vi "Inner Measure.vi"(8 "error in (no error)":errorcluster, 11 "Measurement3D in":refnum<class "Measurement3D.lvclass">) -> (0 "error out":errorcluster, 1 "Current Value":dbl, 2 "Result":dbl, 3 "Measurement3D out":refnum<class "Measurement3D.lvclass">)   [LabVIEW 2014, in "Measurement3D.lvclass"]
uses:
  Measurement3D.lvclass
  Instrument/Instrument/Instrument.lvclass
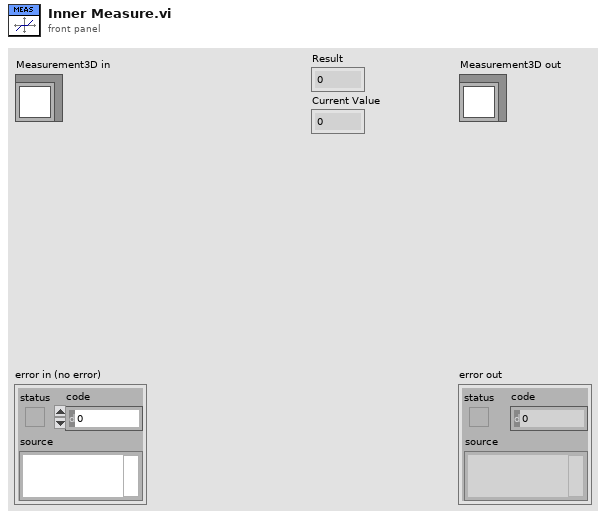
[diagram p1: front panel]
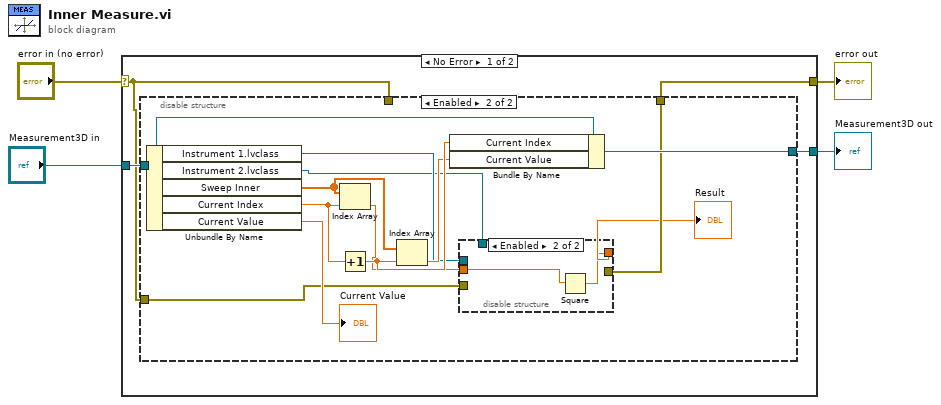
[diagram p0: block diagram]
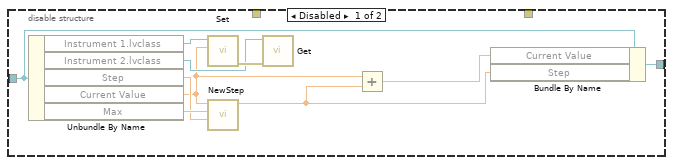
[diagram p2: hidden frame]
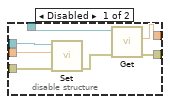
[diagram p3: hidden frame]
diagram:
  n1 = case shown="No Error" "error in (no error)" {
    selector: "error in (no error)" -> [w5 w42]
    tunnel: [w6 w42] -> w3
    tunnel: [w7 w41] -> w1
    tunnel: "Measurement3D in" -> [w8 w41]
    frame No Error {
      n2 = disable-structure shown="Enabled" {
        disable-tunnel: w8 -> [w12 w26]
        disable-tunnel: [w9 w25] -> w7
        disable-tunnel: w5 -> [_ _]
        disable-tunnel: [_ w20] -> w6
        disable-tunnel: w5 -> [_ w24]
        frame Disabled {
          n3 = Unbundle By Name(w12) -> ("Instrument 1.lvclass"=w18:refnum<class "Instrument.lvclass">, "Instrument 2.lvclass"=w14:refnum<class "Instrument.lvclass">, "Step"=w15:dbl, "Current Value"=w13:dbl, "Max"=w16:dbl)
          n4 = call-dynamic "Set.vi"("Numeric"=w13, "Instrument in"=w18) -> ("error out"=w17:errorcluster)  [unwired: 8 in, 1 out]
          n5 = call "NewStep.vi"("Step"=w15, "Max"=w16, "Current Value"=w13) -> ("Step 2"=w10:dbl)  [unwired: 8 in]
          n6 = call-dynamic "Get.vi"("error in (no error)"=w17, "Instrument in"=w14) -> ()  [unwired: 7 in, 3 out]
          n7 = Add(x=w13, y=w10) -> (x+y=w11:dbl)
          n8 = Bundle By Name(cluster=w12, "Current Value"=w11, "Step"=w10) -> (w9:refnum<class "Measurement3D.lvclass">)
        }
        frame Enabled {
          n9 = Unbundle By Name(w26) -> ("Instrument 1.lvclass"=w22:refnum<class "Instrument.lvclass">, "Instrument 2.lvclass"=w21:refnum<class "Instrument.lvclass">, "Sweep Inner"=w29:dbl[], "Current Index"=w30:dbl, "Current Value"=→"Current Value":dbl)
          n10 = Index Array(array=w29, index=w30) -> (element=w23:dbl)
          n11 = Increment(x=w30) -> (x+1=w28:dbl)
          n12 = Index Array(array=w29, index=w28) -> (element=w27:dbl)
          n13 = Bundle By Name(cluster=w26, "Current Index"=w28, "Current Value"=w27) -> (w25:refnum<class "Measurement3D.lvclass">)
          n14 = disable-structure shown="Enabled" {
            disable-tunnel: w24 -> [w38 _]
            disable-tunnel: w23 -> [w37 w40]
            disable-tunnel: w22 -> [w36 _]
            disable-tunnel: w21 -> [w34 _]
            disable-tunnel: [w33 _] -> w20
            disable-tunnel: [w32 w39] -> w19
            frame Disabled {
              n15 = call-dynamic "Set.vi"("error in (no error)"=w38, "Numeric"=w37, "Instrument in"=w36) -> ("error out"=w35:errorcluster)  [unwired: 7 in, 1 out]
              n16 = call-dynamic "Get.vi"("error in (no error)"=w35, "Instrument in"=w34) -> ("error out"=w33:errorcluster, "Numeric"=w32:dbl)  [unwired: 7 in, 1 out]
            }
            frame Enabled {
              n17 = Square(x=w40) -> (x^2=w39:dbl)
            }
          }
          "Result" <- w19
        }
      }
    }
    frame Error {
    }
  }
  "error out" <- w3
  "Measurement3D out" <- w1
